vi "GetType.vi"(8 "error in (no error)":errorcluster, 11 "Configure Edge Trigger Source Msg":refnum<class "Configure Edge Trigger Source Msg.lvclass">) -> (0 "error out":errorcluster, 2 "Data Sample":variant, 3 "Configure Edge Trigger Source Msg":refnum<class "Configure Edge Trigger Source Msg.lvclass">)   [LabVIEW 2014, in "CS++Scope.lvlib" / "Configure Edge Trigger Source Msg.lvclass"]
uses:
  Configure Edge Trigger Source Msg.lvclass
  Configure Edge Trigger Source Msg.lvclass/Configure Edge Trigger Source Msg.ctl
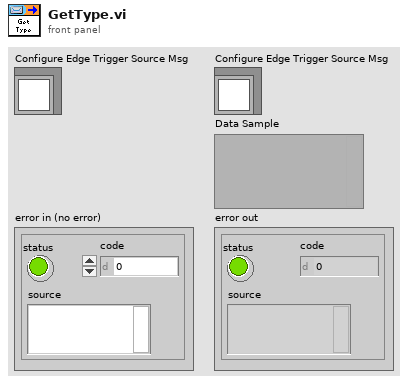
[diagram p1: front panel]
types:
  T1 = cluster{"trigger source (CHANNEL1)":string, "trigger slope (Positive)":i32, "trigger level  (0.0 V)":dbl[unit]}
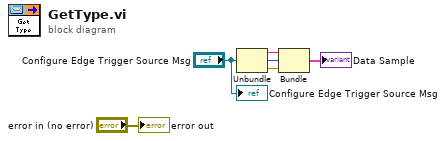
[diagram p0: block diagram]
diagram:
  n1 = Unbundle("Configure Edge Trigger Source Msg") -> (w3:string, w2:i32, w1:dbl[unit])
  n2 = Bundle("trigger source (CHANNEL1)"=w3, "trigger slope (Positive)"=w2, "trigger level  (0.0 V)"=w1) -> (→"Data Sample":T1)  [unwired: 1 in]
  "error out" <- "error in (no error)"
  "Configure Edge Trigger Source Msg" <- "Configure Edge Trigger Source Msg"
